vi "LS 336 T Ramp Text In.vi"(1 "command text in":string[](array[string])=["N/A", "Magent PS", "N/A", "Set Field", "Set Field to 2.0000E+0 @ 0.0000T /min, no wait , extra 0 sec wait", "N/A", "N/A", "", "1", "0", "N/A", "2.000000", "0.000000", "N/A", "N/A", "N/A", "N/A", "N/A", "N/A", "N/A", "N/A", "N/A", "N/A", "N/A", "N/A", "N/A", "N/A", "N/A", "N/A", "N/A", "N/A", "N/A", "N/A", "N/A"]) -> (0 "Timed Ramp":T1={"VISA Resource Name"="", "extra wait"=1, "start"=1.0, "end"=4.0, "Sweep Time (H:M:S)"=10.0, "Log Linear"=FALSE, "Heater Range"=enum."OFF", "Loop"=FALSE} {"Sweep Time (H:M:S)" format="%<%H:%M:%S>t"; "extra wait" min=0; "start" format="%#.7e"; "end" format="%#.7e"})   [LabVIEW 2025]
doc: "Author: Scott Hannahs <sth@magnet.fsu.edu>\n\nThis software is licensed for use under the “MIT License\"\nCopyright (c) 2025 Scott Hannahs, sth@sth@magnet.sthnet.net\n\nPermission is hereby granted, free of charge, to any person obtaining a copy of this software and associated documentation files (the \"Software\"), to deal in the Software without restriction, including without limitation the rights to use, copy, modify, merge, publish, distribute, sublicense, and/or sell copies of the Software, and to permit persons to whom the Software is furnished to do so, subject to the following conditions: The above copyright notice and this permission notice shall be included in all copies or substantial portions of the Software.\n\nTHE SOFTWARE IS PROVIDED \"AS IS\", WITHOUT WARRANTY OF ANY KIND, EXPRESS OR IMPLIED, INCLUDING BUT NOT LIMITED TO THE WARRANTIES OF MERCHANTABILITY, FITNESS FOR A PARTICULAR PURPOSE AND NONINFRINGEMENT. IN NO EVENT SHALL THE AUTHORS OR COPYRIGHT HOLDERS BE LIABLE FOR ANY CLAIM, DAMAGES OR OTHER LIABILITY, WHETHER IN AN ACTION OF CONTRACT, TORT OR OTHERWISE, ARISING FROM, OUT OF OR IN CONNECTION WITH THE SOFTWARE OR THE USE OR OTHER DEALINGS IN THE SOFTWARE."
uses:
  LS 336 T Ramp.ctl
panel:
  out "Numeric":i32
  # "LS 336 Temp Setpoint (K) Ramp"
  # "Log"
  # "End Temp (K)"
  # "Sweep Time (HH:MM:SS)"
  # "Start Temp (K)"
  # "Linear"
  # "seconds"
  # "AND wait extra"
  # "Which Heater to control?"
  # "VISA Name"
  # "Loop 2\n(Probe / 3He Pot)"
  # "Heater Range"
  # "Loop 1\n(Sorb / VTI)"
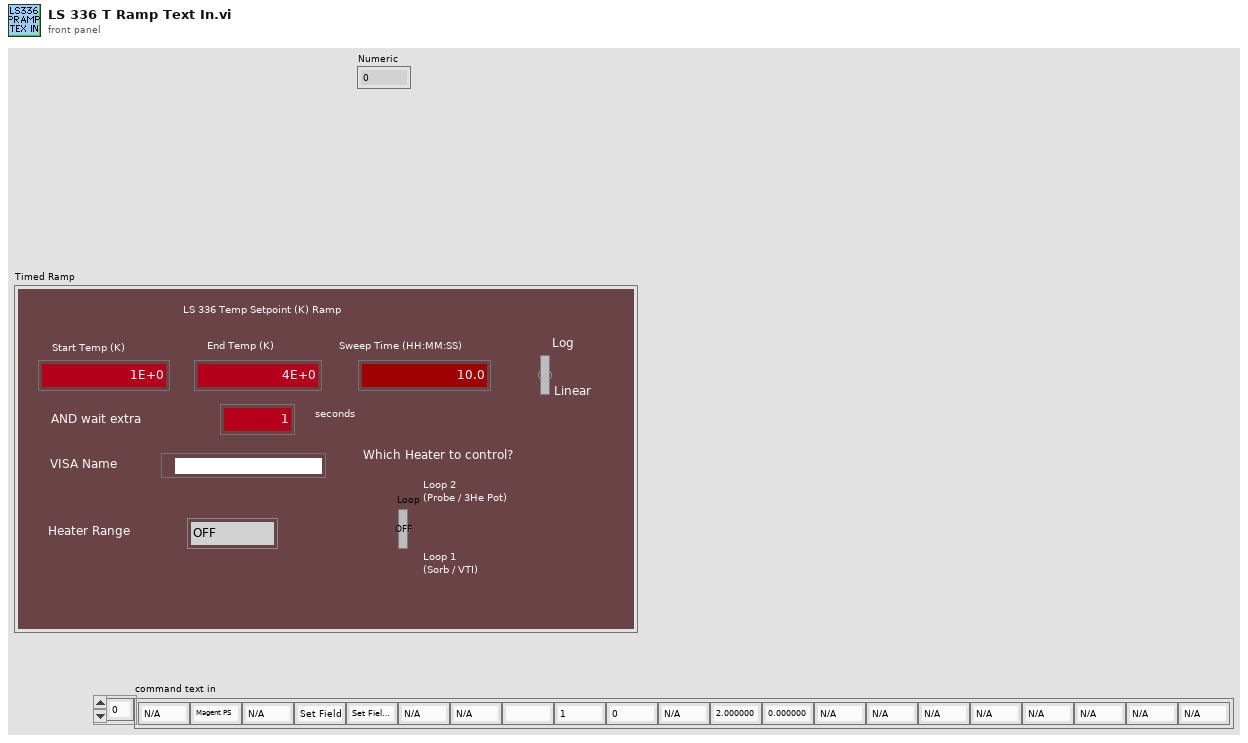
[diagram p1: front panel]
types:
  T1 = typedef "LS 336 T Ramp.ctl" = cluster{"VISA Resource Name":refnum<visa-resource-name>, "extra wait":i32, "start":dbl, "end":dbl, "Sweep Time (H:M:S)":dbl, "Log Linear":bool, "Heater Range":enum16{"OFF", "LOW", "MEIDUM", "HIGH"}, "Loop":bool}
  T2 = cluster{"command text in[0]":string, "command text in[1]":string, "command text in[2]":string, "command text in[3]":string, "command text in[4]":string, "command text in[5]":string, "command text in[6]":string, "command text in[7]":string, "command text in[8]":string, "command text in[9]":string, "command text in[10]":string, "command text in[11]":string, "command text in[12]":string, "command text in[13]":string, "command text in[14]":string, "command text in[15]":string, "command text in[16]":string, "command text in[17]":string, "command text in[18]":string, "command text in[19]":string}
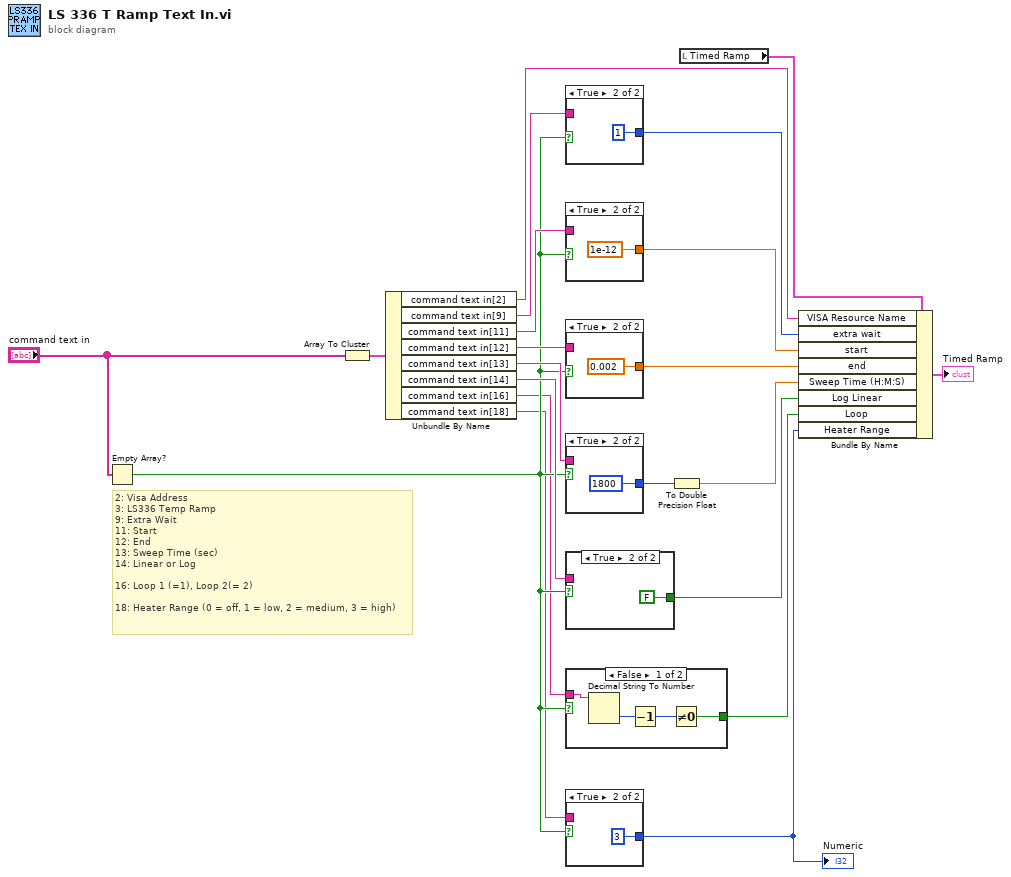
[diagram p0: block diagram]
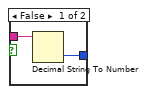
[diagram p2: hidden frame]
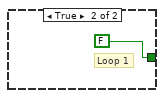
[diagram p3: hidden frame]
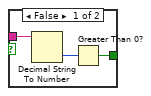
[diagram p4: hidden frame]
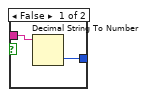
[diagram p5: hidden frame]
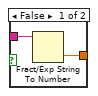
[diagram p6: hidden frame]
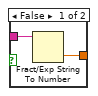
[diagram p7: hidden frame]
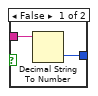
[diagram p8: hidden frame]
diagram:
  # "2: Visa Address\n3: LS336 Temp Ramp\n9: Extra Wait\n11: Start\n12: End\n13: Sweep Time (sec)\n14: Linear or Log\n\n16: Loop 1 (=1), Loop 2(= 2)\n\n18: Heater Range (0 = off, 1 = low, 2 = medium, 3 = high)"
  n1 = Empty Array?(array="command text in") -> (empty?=w7:bool)
  n2 = Array To Cluster(array="command text in") -> (cluster=w21:T2)
  n3 = Unbundle By Name(w21) -> ("command text in[2]"=w19:string, "command text in[9]"=w18:string, "command text in[11]"=w16:string, "command text in[12]"=w14:string, "command text in[13]"=w12:string, "command text in[14]"=w9:string, "command text in[16]"=w5:string, "command text in[18]"=w4:string)
  n4 = case shown="True" w7 {
    tunnel: w18 -> [w23 _]
    tunnel: [w22 u16 1 ("Value (Signaling)")] -> w17
    frame False {
      n5 = Decimal String To Number(string=w23) -> (number=w22:i32)  [unwired: 2 in, 1 out]
    }
    frame True {
    }
  }
  n6 = case shown="True" w7 {
    tunnel: [w26 1e-12] -> w15
    tunnel: w16 -> [w25 _]
    frame False {
      n7 = Fract/Exp String To Number(string=w25) -> (number=w26:dbl)  [unwired: 3 in, 1 out]
    }
    frame True {
    }
  }
  n8 = case shown="True" w7 {
    tunnel: [w29 0.002] -> w13
    tunnel: w14 -> [w28 _]
    frame False {
      n9 = Fract/Exp String To Number(string=w28) -> (number=w29:dbl)  [unwired: 3 in, 1 out]
    }
    frame True {
    }
  }
  n10 = case shown="True" w7 {
    tunnel: w12 -> [w32 _]
    tunnel: [w31 1800] -> w11
    frame False {
      n11 = Decimal String To Number(string=w32) -> (number=w31:i32)  [unwired: 2 in, 1 out]
    }
    frame True {
    }
  }
  n12 = case shown="True" w7 {
    tunnel: w9 -> [w36 _]
    tunnel: [w35 FALSE] -> w8
    frame False {
      n13 = Decimal String To Number(string=w36) -> (number=w34:i32)  [unwired: 2 in, 1 out]
      n14 = Greater Than 0?(x=w34) -> (x > 0?=w35:bool)
    }
    frame True {
    }
  }
  n15 = case shown="False" w7 {
    tunnel: [w39 FALSE] -> w6
    tunnel: w5 -> [w38 _]
    frame False {
      n16 = Decimal String To Number(string=w38) -> (number=w41:i32)  [unwired: 2 in, 1 out]
      n17 = Decrement(x=w41) -> (x-1=w40:i32)
      n18 = Not Equal To 0?(x=w40) -> (x != 0?=w39:bool)
    }
    frame True {
      # "Loop 1"
    }
  }
  n19 = case shown="True" w7 {
    tunnel: w4 -> [w44 _]
    tunnel: [w43 3] -> w3
    frame False {
      n20 = Decimal String To Number(string=w44) -> (number=w43:i32)  [unwired: 2 in, 1 out]
    }
    frame True {
    }
  }
  "Numeric" <- w3
  n21 = To Double Precision Float(number=w11) -> (double precision float=w10:dbl)
  n22 = local read "Timed Ramp"() -> (w2:T1)
  n23 = Bundle By Name(cluster=w2, "VISA Resource Name"=w19, "extra wait"=w17, "start"=w15, "end"=w13, "Sweep Time (H:M:S)"=w10, "Log Linear"=w8, "Loop"=w6, "Heater Range"=w3) -> (→"Timed Ramp":T1)
